vi "Simple Bluetooth - Server.vi"() -> ()   [LabVIEW 2016]
doc: "Demonstrates how to set up a basic Bluetooth connection, send data to the specified channel once a connection has been established, and terminate the connection once the data has been sent. This VI is designed to stop if the Bluetooth connection is terminated. The data sent in this example is an array of random numbers."
panel:
  in  "Offset":dbl(slide) scale=-10.0..10.0
  in  "Amplitude":dbl(slide) scale=0.0..10.0
  out "Data Transimtted":string
  in  "Client Closed":string="The client VI closed the connection."
  out "Waveform Graph":dbl[](graph)
  out "Address":string
  out "Channel":u16
  in  "Stop":bool
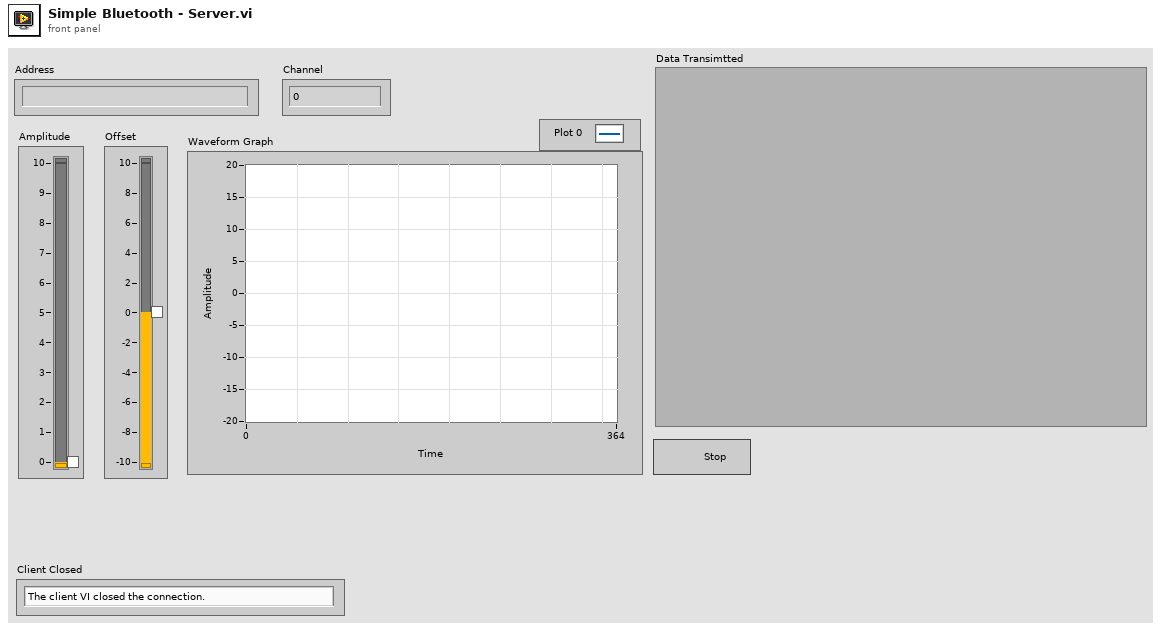
[diagram p1: front panel]
types:
  T1 = cluster{"Address":string, "Device Name":string}[]
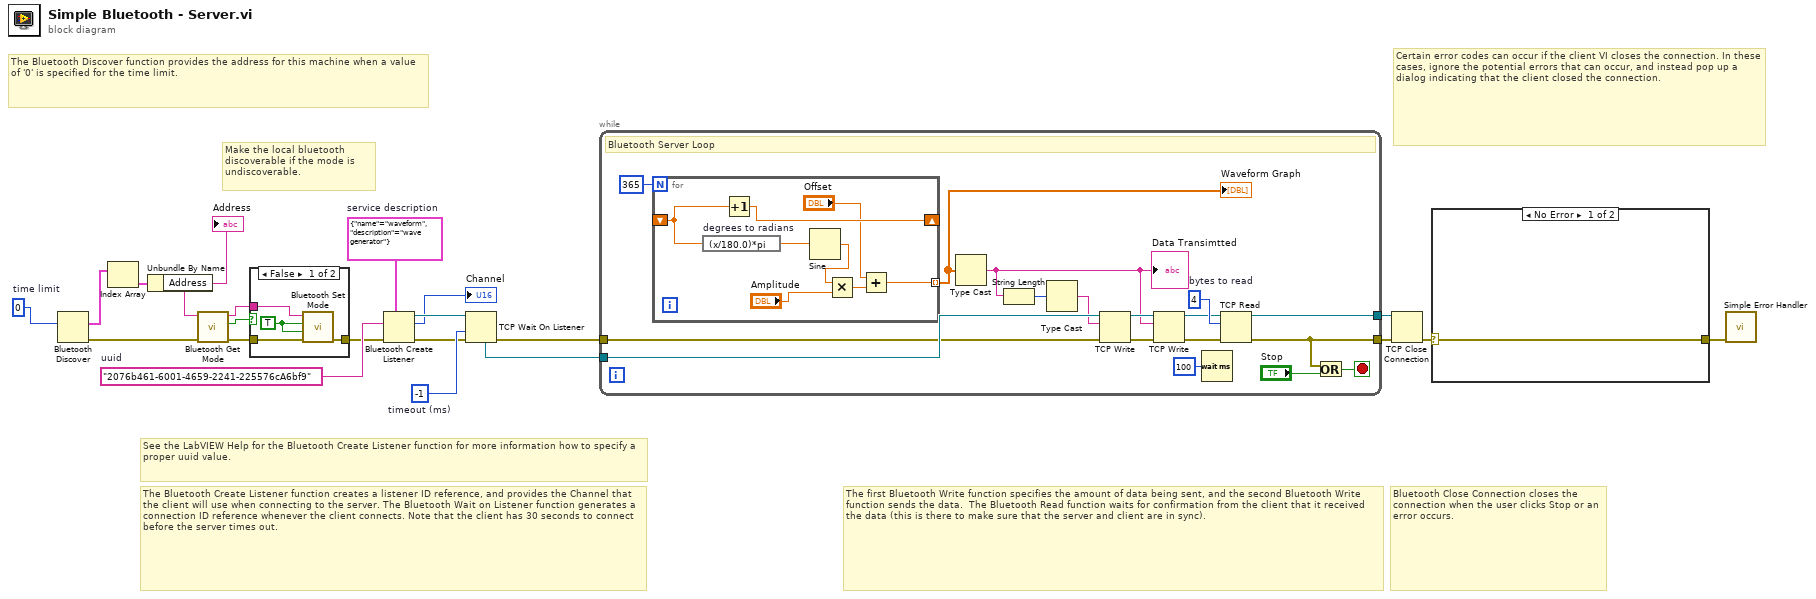
[diagram p0: block diagram]
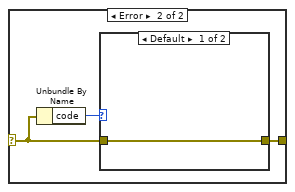
[diagram p3: hidden frame]
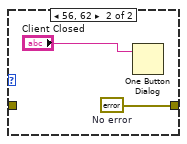
[diagram p4: hidden frame]
diagram:
  w11 = cluster{"name":string, "description":string} {"name"="waveform", "description"="wave generator"}  # service description
  w14 = -1  # timeout (ms)
  w10 = "2076b461-6001-4659-2241-225576cA6bf9"  # uuid
  w17 = 0  # time limit
  # "Make the local bluetooth discoverable if the mode is undiscoverable."
  # "See the LabVIEW Help for the Bluetooth Create Listener function for more information how to specify a proper uuid value."
  # "Bluetooth Close Connection closes the connection when the user clicks Stop or an error occurs."
  # "The Bluetooth Create Listener function creates a listener ID reference, and provides the Channel that the client will use when connecting to the server. The Bluetooth Wait on Listener function generates a connection ID reference whenever the client connects. Note that the client has 30 seconds to connect before the server times out."
  # "The Bluetooth Discover function provides the address for this machine when a value of '0' is specified for the time limit."
  # "Certain error codes can occur if the client VI closes the connection. In these cases, ignore the potential errors that can occur, and instead pop up a dialog indicating that the client closed the connection."
  # "The first Bluetooth Write function specifies the amount of data being sent, and the second Bluetooth Write function sends the data.  The Bluetooth Read function waits for confirmation from the client that it received the data (this is there to make sure that the server and client are in sync)."
  n1 = Bluetooth Discover(10:w17) -> (0:w5:errorcluster, 2:w16:T1)  [unwired: 1 in, 1 out]
  n2 = Index Array(array=w16) -> (element=w15:cluster{"Address":string, "Device Name":string})  [unwired: 1 in]
  n3 = Unbundle By Name(w15) -> ("Address"=w2:string)
  "Address" <- w2
  n4 = call <vilib>:"Bluetooth Get Mode.vi"("error in (no error)"=w5, "address in"=w2) -> ("error out"=w4:errorcluster, "discoverable"=w3:bool, "address out"=w1:string)  [unwired: 2 in, 1 out]
  n5 = case shown="False" w3 {
    tunnel: [w24 w26] -> w6
    tunnel: w4 -> [w23 w26]
    tunnel: w1 -> [w22 _]
    frame False {
      w25 = TRUE ("discoverable")
      n6 = call <vilib>:"Bluetooth Set Mode.vi"("error in (no error)"=w23, "connectable"=w25, "discoverable"=w25, "address in"=w22) -> ("error out"=w24:errorcluster)  [unwired: 2 in, 1 out]
    }
    frame True {
    }
  }
  n7 = Bluetooth Create Listener(6:w11, 8:w6, 10:w10) -> (0:w7:errorcluster, 2:→"Channel":u16, 3:w19:refnum<k31>)  [unwired: 1 out]
  n8 = TCP Wait On Listener(8:w7, 9:w14, 11:w19) -> (0:w12:errorcluster, 4:w13:refnum<k31>)  [unwired: 4 out]
  n9 = while {
    tunnel: [w27] -> w20
    tunnel: [w28] -> w21
    tunnel: w13 -> [w43]
    tunnel: w12 -> [w34]
    stop <- w36 stop-if-true
    w31 = 4  # bytes to read
    # "Bluetooth Server Loop"
    n10 = for {
      N: 365 ("# of Points") -> [_]
      tunnel: [w45] -> w32 mode=indexing
      shift-right: [w50] -> _
      shift-left: _ -> [w51]
      n11 = expression code="(x/180.0)*pi" "degrees to radians"(w51) -> (w48:dbl)
      n12 = Increment(x=w51) -> (x+1=w50:dbl)
      n13 = Sine(x=w48) -> (sin(x)=w44:dbl)
      n14 = Multiply(x=w44, y="Amplitude") -> (x*y=w47:dbl)
      n15 = Add(x="Offset", y=w47) -> (x+y=w45:dbl)
    }
    "Waveform Graph" <- w32
    n16 = Type Cast(x=w32) -> (*(type *) &x=w38:string)  [unwired: 1 out]
    "Data Transimtted" <- w38
    n17 = String Length(string=w38) -> (length=w40:i32)
    n18 = Type Cast(x=w40) -> (*(type *) &x=w39:string)  [unwired: 1 out]
    n19 = TCP Write(connection ID=w43, data in=w39, error in (no error)=w34) -> (connection ID out=w42:refnum<k31>, error out=w41:errorcluster)  [unwired: 2 out]
    n20 = TCP Write(connection ID=w42, data in=w38, error in (no error)=w41) -> (connection ID out=w30:refnum<k31>, error out=w29:errorcluster)  [unwired: 2 out]
    n21 = Wait (ms)(milliseconds to wait=u32 100) -> ()  [unwired: 1 out]
    n22 = TCP Read(connection ID=w30, bytes to read=w31, error in (no error)=w29) -> (connection ID out=w28:refnum<k31>, error out=w27:errorcluster)  [unwired: 3 out]
    n23 = Or(x=w27, y="Stop") -> (x .or. y?=w36:bool)
  }
  n24 = TCP Close Connection(connection ID=w21, error in (no error)=w20) -> (error out=w9:errorcluster)  [unwired: 2 out]
  n25 = case shown="No Error" w9 {
    selector: w9 -> [w52 w54]
    tunnel: [w52 w53] -> w8
    frame No Error {
    }
    frame Error {
      n26 = Unbundle By Name(w54) -> ("code"=w55:i32)
      n27 = case shown="Default" w55 {
        tunnel: w54 -> [w56 _]
        tunnel: [w56 w58] -> w53
        frame Default {
        }
        frame 56, 62 {
          w58 = errorcluster {"status"=FALSE, "code"=0, "source"=""}  # No error
          n28 = One Button Dialog(message="Client Closed") -> ()  [unwired: 1 in, 1 out]
        }
      }
    }
  }
  n29 = call <vilib>:"Simple Error Handler.vi"("error in (no error)"=w8) -> ()  [unwired: 1 in, 8 out]
